vi "Overall_system_A0.vi"() -> ()   [LabVIEW 2019]
doc: "This VI is th overall VI that can read the weight, rfid and camera (and save the data into a csv file). When certain threshold are met it can also send a telegram message at the end."
uses:
  Program Files (x86)/National Instruments/LabVIEW 2019/examples/Instrument IO/Serial/support/Serial - Settings.ctl
  dependencies/notification/Telegram-Bot-master (1)/Telegram-Bot-master/Telegram/Methods/TypeDefs/SendMessageType.ctl
panel:
  in  "start rfid (debug)":bool
  out "RFID Check":string
  out "Weight":string
  in  "Serial Settings":T1={"baud rate"=9600, "data bits"=8, "parity"=enum."None", "stop bits"=10, "flow control"=0} {"flow control" items=["None"=0, "XON/XOFF"=1, "RTS/CTS"=2, "DTR/DSR"=4]; "stop bits" items=["1.0"=10, "1.5"=15, "2.0"=20]; "data bits" min=5 max=8 step=1; "baud rate" items=["75"=75, "110"=110, "134"=134, "150"=150, "300"=300, "600"=600, "1200"=1200, "1800"=1800, "2400"=2400, "4800"=4800, "7200"=7200, "9600"=9600, "14400"=14400, "19200"=19200, "28800"=28800, "38400"=38400, "56000"=56000, "57600"=57600, "115200"=115200, "128000"=128000, "230400"=230400]}
  in  "delay before read (ms)":u32=500
  in  "Weight VISA resource name":refnum<visa-resource-name>="COM1"
  in  "RFID":string
  in  "Start camera (debug)":bool
  out "Health Monitoring in Progress":bool
  in  "Bird is underfeeding (debug)":bool
  out "Current image":T2(plugin-control)
  in  "Camera Name":refnum<k21>="cam0" caption="IMAQdx Session"
  # "Intelligent Health Monitoring System"
  # "grams"
  # "Weight detection settings:"
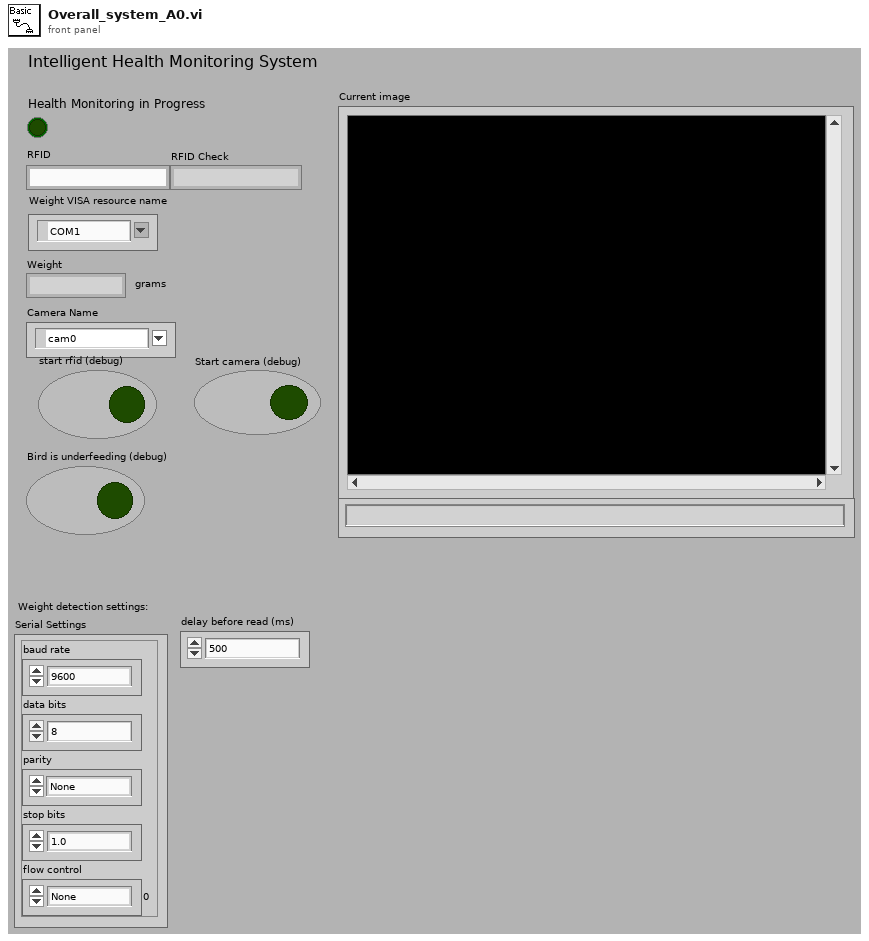
[diagram p1: front panel]
types:
  T1 = typedef "Serial - Settings.ctl" = cluster{"baud rate":u32, "data bits":u16, "parity":enum16{"None", "Odd", "Even", "Mark", "Space"}, "stop bits":u16, "flow control":u16}
  T2 = typedef "IMAQ Image.ctl" = refnum<image>
  T3 = typedef "SendMessageType.ctl" = enum16{"Text", "ReplyKeyboardMarkup", "ReplyKeyboardRemove"}
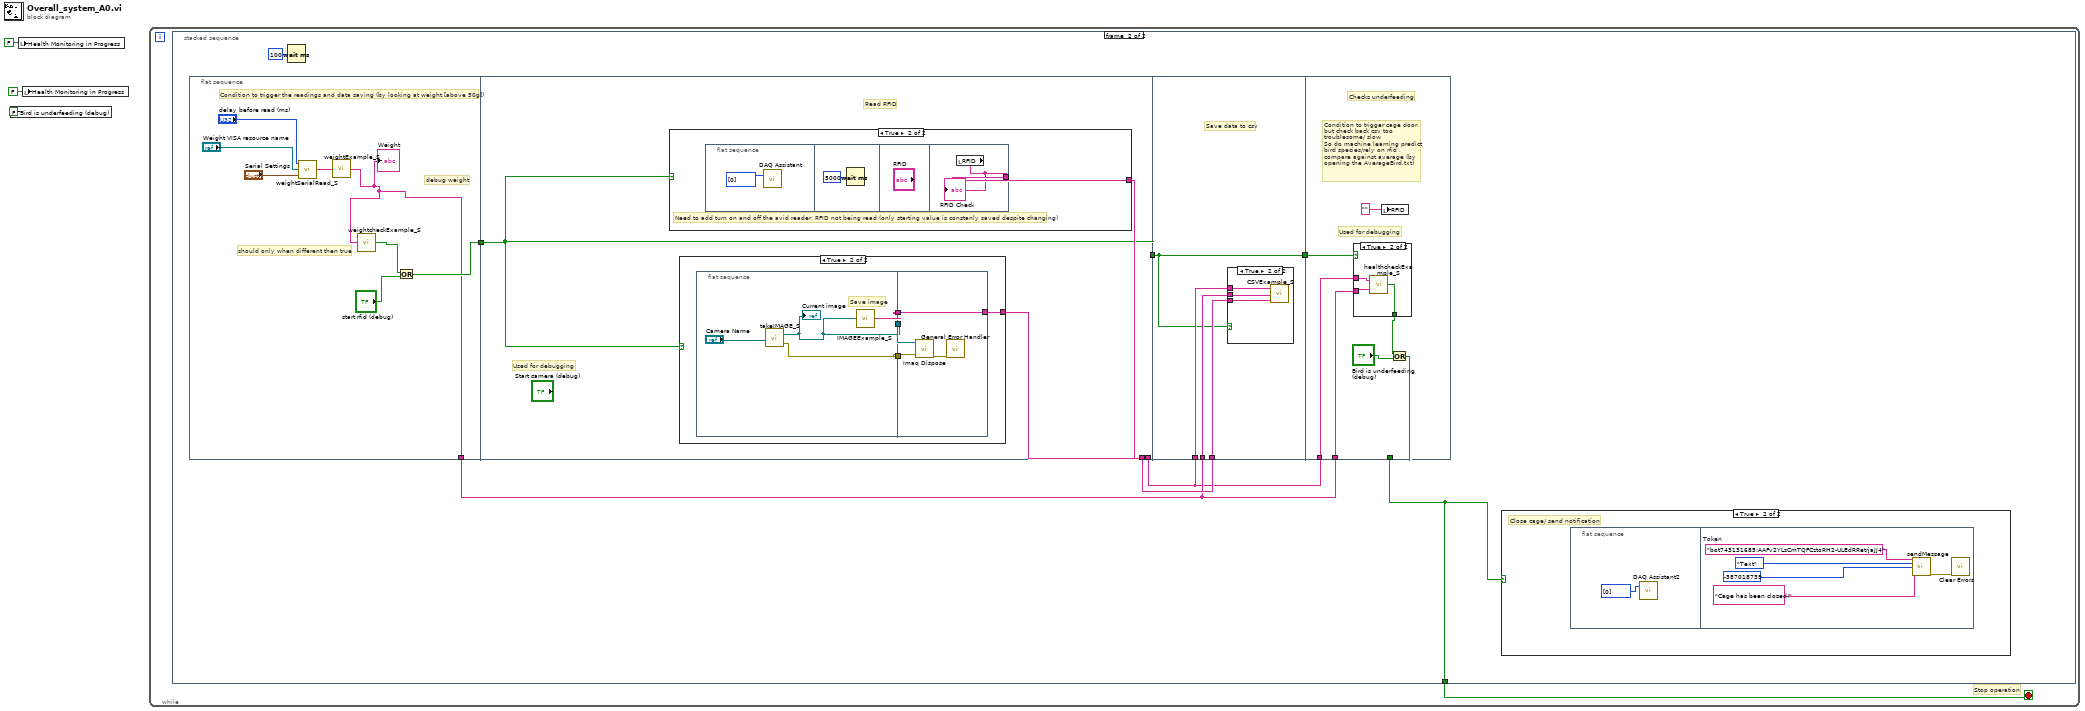
[diagram p0: block diagram]
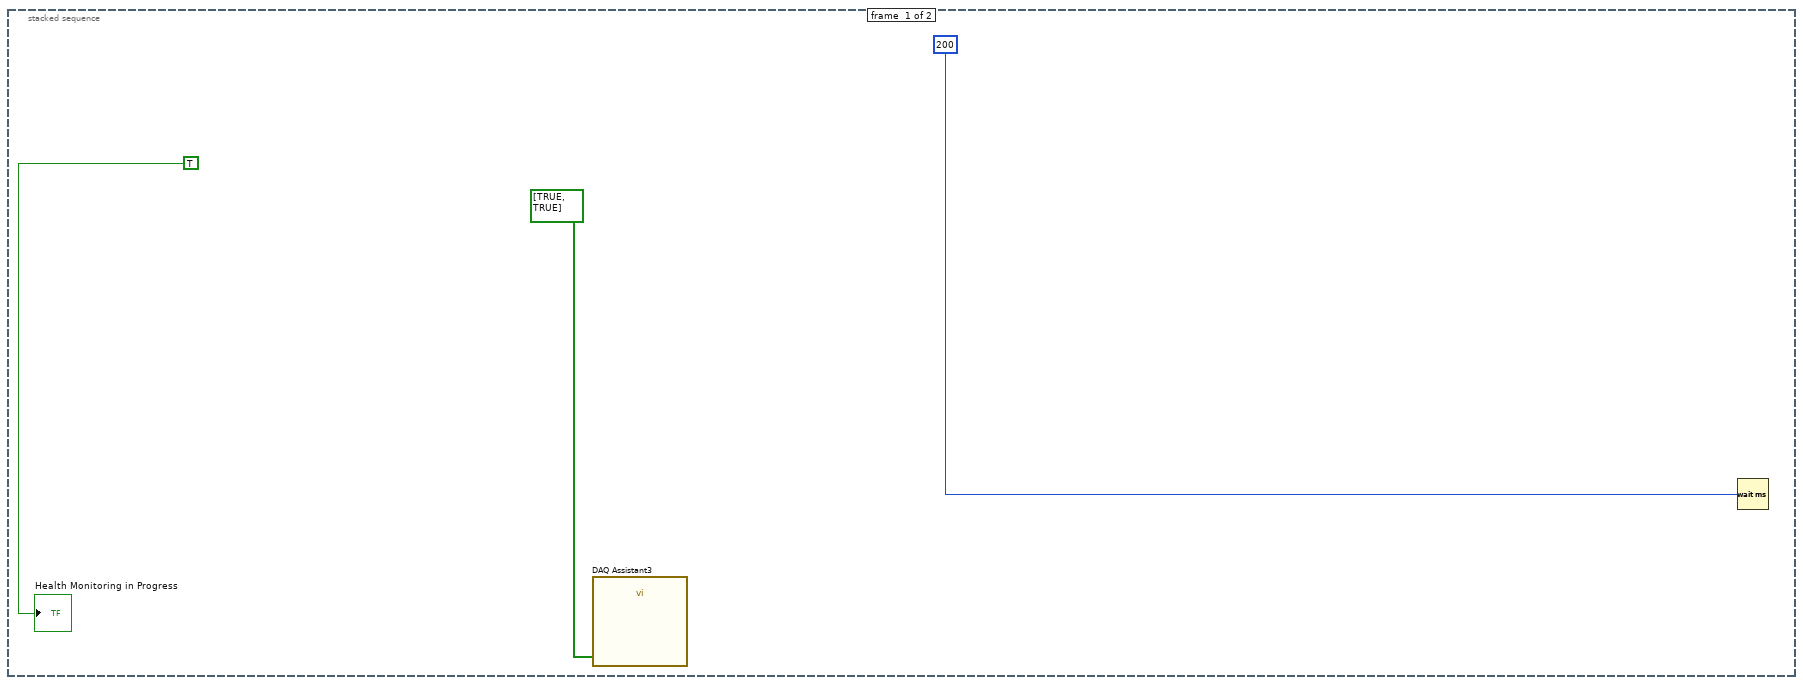
[diagram p2: hidden frame]
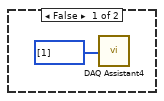
[diagram p4: hidden frame]
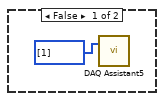
[diagram p7: hidden frame]
diagram:
  n1 = local write "Bird is underfeeding (debug)"(FALSE ("Bird is underfeeding")) -> ()
  n2 = local write "Health Monitoring in Progress"(FALSE ("Health Monitoring in Progress")) -> ()
  n3 = local write "Health Monitoring in Progress"(FALSE ("Health Monitoring in Progress")) -> ()
  n4 = while {
    stop <- w4 stop-if-true
    # "Stop operation"
    n5 = stacked-sequence {
      tunnel: [_ w14] -> w4
      frame #0 {
        n6 = call "DAQ Assistant3"("data"=bool[] [TRUE, TRUE]) -> ()  [unwired: 17 in, 2 out]
        n7 = Wait (ms)(milliseconds to wait=u32 200) -> ()  [unwired: 1 out]
        "Health Monitoring in Progress" <- TRUE ("Health Monitoring in Progress")
      }
      frame #1 {
        n8 = flat-sequence {
          tunnel: [w16] -> w9
          tunnel: [w22] -> w13
          tunnel: [w26] -> w8
          tunnel: [w25] -> w10
          tunnel: w13 -> [w24]
          tunnel: [w24] -> w12
          tunnel: w12 -> [w44]
          tunnel: [w44] -> w11
          tunnel: w10 -> [w47]
          tunnel: w9 -> [w46]
          tunnel: w8 -> [w45]
          tunnel: [w52] -> w14
          tunnel: w9 -> [w57]
          tunnel: w11 -> [w56]
          tunnel: w8 -> [w55]
          frame #0 {
            # "debug weight"
            # "Condition to trigger the readings and data saving (by looking at weight [above 50g])"
            # "should only when different then true"
            n9 = call "weightSerialRead_S.vi"("Serial Settings"="Serial Settings", "Weight VISA resource name"="Weight VISA resource name", "delay before read (ms)"="delay before read (ms)") -> ("String"=w17:string)
            n10 = call "weightExample_S.vi"("weight"=w17) -> ("String"=w16:string)
            "Weight" <- w16
            n11 = call "weightcheckExample_S.vi"("weight"=w16) -> ("Boolean"=w21:bool)
            n12 = Or(x=w21, y="start rfid (debug)") -> (x .or. y?=w22:bool)
          }
          frame #1 {
            # "Used for debugging"
            # "Read RFID"
            n13 = case shown="True" w24 {
              tunnel: [_ w40] -> w26
              frame False {
                n14 = call "DAQ Assistant4"("data"=u32[] [1]) -> ()  [unwired: 17 in, 2 out]
              }
              frame True {
                # "Need to add turn on and off the avid reader, RFID not being read (only starting value is constanly saved despite changing)"
                n15 = flat-sequence {
                  tunnel: [w43] -> w40
                  frame #0 {
                    n16 = call "DAQ Assistant"("data"=u32[] [0]) -> ()  [unwired: 17 in, 2 out]
                  }
                  frame #1 {
                    n17 = Wait (ms)(milliseconds to wait=u32 5000) -> ()  [unwired: 1 out]
                  }
                  frame #2 {
                  }
                  frame #3 {
                    n18 = local read "RFID"() -> (w43:string)
                    "RFID Check" <- w43
                  }
                }
              }
            }
            n19 = case shown="True" w24 {
              tunnel: [_ w28] -> w25
              frame False {
              }
              frame True {
                n20 = flat-sequence {
                  tunnel: [w32] -> w30
                  tunnel: [w31] -> w29
                  tunnel: [w34] -> w27
                  tunnel: w30 -> [w38]
                  tunnel: w29 -> [w36]
                  tunnel: [w35] -> w28
                  tunnel: w27 -> [w35]
                  frame #0 {
                    # "Save image"
                    n21 = call "takeIMAGE_S.vi"("Camera Name"="Camera Name") -> ("Current image"=w31:T2, "error in (no error)"=w32:errorcluster)
                    "Current image" <- w31
                    n22 = call "IMAGEExample_S.vi"("Image"=w31) -> ("String"=w34:string)
                  }
                  frame #1 {
                    n23 = call "Imaq Dispose"("Image"=w36, "error in (no error)"=w38) -> ("error out"=w37:errorcluster)  [unwired: 4 in]
                    n24 = call <vilib>:"General Error Handler.vi"("error in (no error)"=w37) -> ()  [unwired: 2 in, 13 out]
                  }
                }
              }
            }
          }
          frame #2 {
            # "Save data to csv"
            n25 = case shown="True" w44 {
              tunnel: w47 -> [_ w48]
              tunnel: w46 -> [_ w49]
              tunnel: w45 -> [_ w50]
              frame False {
              }
              frame True {
                n26 = call "CSVExample_S.vi"("imageId"=w48, "weight"=w49, "rfid"=w50) -> ()
              }
            }
          }
          frame #3 {
            # "Used for debugging"
            # "Condition to trigger cage door,\nbut check back csv too troublesome/ slow\nSo do machine learning predict bird species/rely on rfid , compare against average (by opening the AverageBird.txt)"
            # "Checks underfeeding"
            n27 = case shown="True" w56 {
              tunnel: [_ w58] -> w54
              tunnel: w55 -> [_ w59]
              tunnel: w57 -> [_ w60]
              frame False {
              }
              frame True {
                n28 = call "healthcheckExample_S.vi"("weight"=w60, "rfid"=w59) -> ("Boolean"=w58:bool)
              }
            }
            n29 = local write "RFID"("") -> ()
            n30 = Or(x=w54, y="Bird is underfeeding (debug)") -> (x .or. y?=w52:bool)
          }
        }
        n31 = Wait (ms)(milliseconds to wait=u32 100) -> ()  [unwired: 1 out]
        n32 = case shown="True" w14 {
          frame False {
            n33 = call "DAQ Assistant5"("data"=u32[] [1]) -> ()  [unwired: 17 in, 2 out]
          }
          frame True {
            # "Close cage/ send notification"
            n34 = flat-sequence {
              frame #0 {
                n35 = call "DAQ Assistant2"("data"=u32[] [0]) -> ()  [unwired: 17 in, 2 out]
              }
              frame #1 {
                w66 = "bot743131685:AAFv2YLsCmTQFCztoRH2-ULEdRRetrjaJJ4"  # Token
                n36 = call "sendMessage.vi"("Token"=w66, "MsgType"=SendMessageType."Text", "ChatId"=i64 -387018739, "Text"="Cage has been closed!") -> ("error out"=w67:errorcluster)  [unwired: 11 in]
                n37 = call <vilib>:"Clear Errors.vi"("error in (no error)"=w67) -> ()  [unwired: 5 in, 2 out]
              }
            }
          }
        }
      }
    }
  }
